vi "Save_persona.vi"(6 "Descrição:":string, 7 "Tipo de eixo dos XX":string, 8 "Time Step:":string, 9 "Nome do utilizador:":string) -> (0 "Descrição:":string, 1 "Tipo de eixo dos XX":string, 2 "Time Step:":string, 3 "Nome do utilizador:":string)   [LabVIEW 2013]
panel:
  in  "Cancel Button":bool
  in  "OK Button":bool
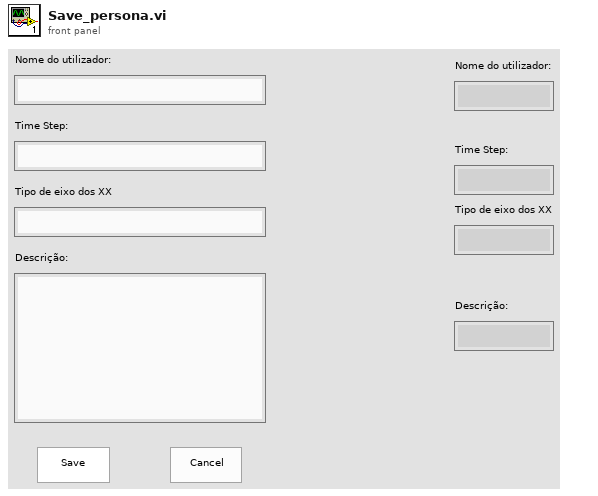
[diagram p1: front panel]
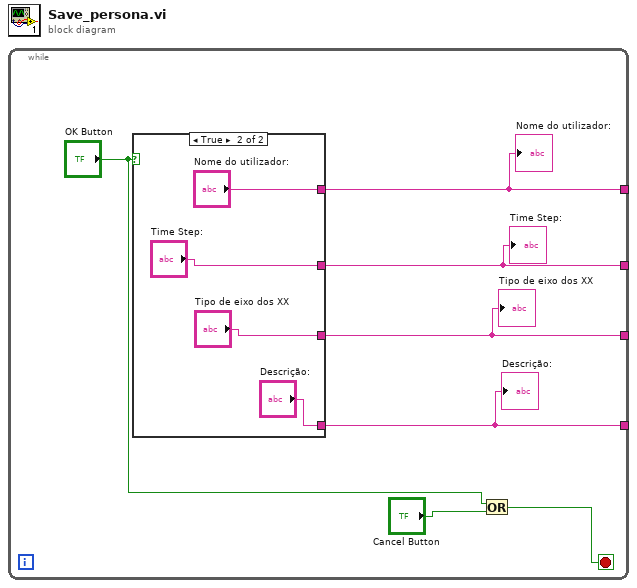
[diagram p0: block diagram]
diagram:
  n1 = while {
    tunnel: [w7] -> _
    tunnel: [w6] -> _
    tunnel: [w5] -> _
    tunnel: [w4] -> _
    stop <- w2 stop-if-true
    n2 = case shown="True" "OK Button" {
      tunnel: [_ "Nome do utilizador:"] -> w7
      tunnel: [_ "Time Step:"] -> w6
      tunnel: [_ "Tipo de eixo dos XX"] -> w5
      tunnel: [_ "Descrição:"] -> w4
      frame False {
      }
      frame True {
      }
    }
    "Nome do utilizador:" <- w7
    "Time Step:" <- w6
    "Tipo de eixo dos XX" <- w5
    "Descrição:" <- w4
    n3 = Or(x="OK Button", y="Cancel Button") -> (x .or. y?=w2:bool)
  }
